vi "OSc_Lock_Unlock.vi"(8 "entrée d'erreur (pas d'erreur)":errorcluster, 10 "Control-Client old entrée":refnum<class "Control-Client.lvclass">, 11 "Control-Client new entrée":refnum<class "Control-Client.lvclass">) -> (0 "sortie d'erreur":errorcluster, 2 "Control-Client old out":refnum<class "Control-Client.lvclass">, 3 "Control-Client new out":refnum<class "Control-Client.lvclass">)   [LabVIEW 2018, in "Control-Client.lvclass"]
uses:
  Control-Client.lvclass
  Control-Client.lvclass/Control-Client.ctl
  controls/Gauge_pump/Gauge_pump.xctl
  dependecies/XControls/CellsDL/ControlDL.xctl
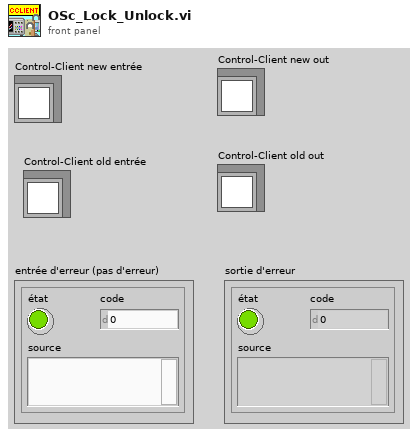
[diagram p1: front panel]
types:
  T1 = enum8{"Enabled", "Disabled", "Disabled and Grayed Out"}
  T2 = typedef "Control-Client.lvclass/Controls-with-permissions_CLIENT.ctl" = cluster{"Server ON/OFF":refnum<vi>, "Detector connect":refnum<vi>, "DL connect":refnum<vi>, "DAQmx connect":refnum<vi>, "All connect":refnum<vi>, "Start measurement":refnum<vi>, "Move Crystal":refnum<vi>, "Relay key heater":refnum<vi>, "Laser Shutter":refnum<vi>, "Accelerator Shutter":refnum<vi>, "Power":refnum<vi>, "Unlock":refnum<vi>, "RT":refnum<vi>, "Faraday Cup":refnum<vi>, "Osc connect":refnum<vi>, "ELYSE pulses":refnum<vi>, "Cells":refnum<vi>, "Pump":refnum<vi>, "# par point":refnum<vi>, "Alarm":refnum<vi>, "oscilloscopeRead":refnum<vi>, "WCM_state":refnum<vi>, "ControlDL":refnum<vi>}
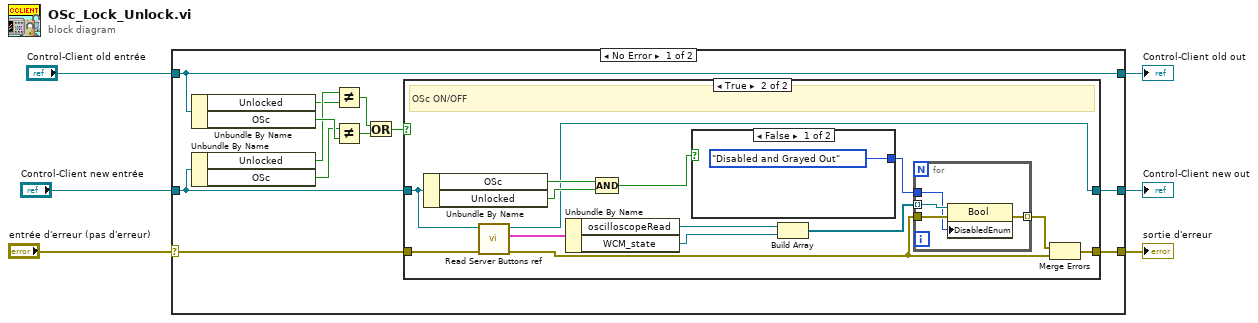
[diagram p0: block diagram]
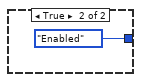
[diagram p3: hidden frame]
diagram:
  n1 = case shown="No Error" "entrée d'erreur (pas d'erreur)" {
    selector: "entrée d'erreur (pas d'erreur)" -> [w9 w41]
    tunnel: [w18 w41] -> w6
    tunnel: "Control-Client new entrée" -> [w17 w42]
    tunnel: "Control-Client old entrée" -> [w7 w43]
    tunnel: [w8 w42] -> w2
    tunnel: [w7 w43] -> w1
    frame No Error {
      n2 = Unbundle By Name(w7) -> ("Unlocked"=w10:bool, "OSc"=w16:bool)
      n3 = Unbundle By Name(w17) -> ("Unlocked"=w14:bool, "OSc"=w15:bool)
      n4 = Not Equal?(x=w14, y=w10) -> (x != y?=w13:bool)
      n5 = Not Equal?(x=w15, y=w16) -> (x != y?=w12:bool)
      n6 = Or(x=w13, y=w12) -> (x .or. y?=w11:bool)
      n7 = case shown="True" w11 {
        tunnel: w17 -> [w19 w31]
        tunnel: [w20 w23] -> w18
        tunnel: w9 -> [w20 w33]
        tunnel: [w19 w21] -> w8
        frame False {
        }
        frame True {
          # "OSc ON/OFF"
          n8 = Unbundle By Name(w31) -> ("OSc"=w30:bool, "Unlocked"=w29:bool)
          n9 = call "Read Server Buttons ref.vi"("error in (no error)"=w33, "Control-Client in"=w31) -> ("error out"=w24:errorcluster, "Server Buttons ref"=w34:T2, "Control-Client out"=w21:refnum<class "Control-Client.lvclass">)  [unwired: 7 in]
          n10 = Unbundle By Name(w34) -> ("oscilloscopeRead"=w28:refnum<vi>, "WCM_state"=w27:refnum<vi>)
          n11 = Compound Arithmetic op=AND(w30, w29) -> (w32:bool)
          n12 = case shown="False" w32 {
            tunnel: [T1."Disabled and Grayed Out" ("Désactivé") T1."Enabled" ("Désactivé")] -> w22
            frame False {
            }
            frame True {
            }
          }
          n13 = Build Array(w28, w27) -> (w26:refnum<vi>[])
          n14 = for {
            tunnel: w26 -> [w38] mode=indexing
            tunnel: w24 -> [w37]
            tunnel: [w36] -> w25 mode=indexing
            tunnel: w22 -> [w35]
            n15 = property class="Bool"(reference=w38, error in=w37, "DisabledEnum"=w35) -> (error out=w36:errorcluster)  [unwired: 1 out]
          }
          n16 = Merge Errors(w25, w24) -> (w23:errorcluster)
        }
      }
    }
    frame Error {
    }
  }
  "sortie d'erreur" <- w6
  "Control-Client new out" <- w2
  "Control-Client old out" <- w1
